vi "1darray.vi"() -> ()   [LabVIEW 2009]
panel:
  out "Array":dbl[](array[numeric])
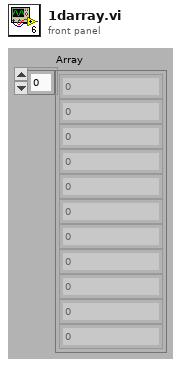
[diagram p1: front panel]
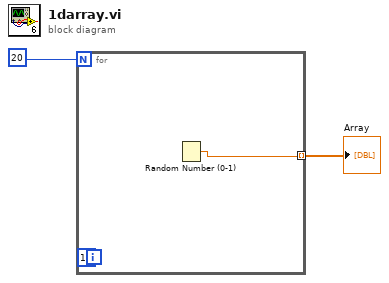
[diagram p0: block diagram]
diagram:
  n1 = for {
    N: 20 -> [_]
    tunnel: [w3] -> w2 mode=indexing
    (unwired) 10
    n2 = Random Number (0-1)() -> (number: 0 to 1=w3:dbl)
  }
  "Array" <- w2
